vi "Write to Lights.vi"   [LabVIEW 2015]
uses:
  Common Code/Shooter State.ctl
  Common Code/Utilities/TimeManager.vi
  Common Code/Change Detect.vi
  Common Code/Change Detect Boolean.vi
  Robot Code/Robot Global Data.vi
types:
  T1 = typedef "Shooter State.ctl" = enum16{"Idle", "Warmup", "Shooter Ready", "Shoot"}
  T2 = typedef "Dashboard Display Data.ctl" = cluster{"Auton Command Cluster":T3, "Auton File Lists":T4, "Drivetrain Status Cluster":T5, "Encoder Values":T8, "IMU Data":T10, "Power and Diagnostic Data":T13, "Gyro":dbl, "Shooter State Cluster":T16, "Intake Status Cluster":T19, "Ultrasonic Data":T22, "Climb Status Cluster":T23, "Loop Times":T25}
  T3 = typedef "Auton Command Cluster.ctl" = cluster{"Command ID":i32, "maxTime":dbl, "Y Distance":dbl, "Heading":dbl, "Throttle":dbl, "Async":dbl, "Velocity":dbl, "Acceleration":dbl, "To":dbl, "Condition":dbl, "Shot Type":dbl, "Left RPM":dbl, "Override RPM":i32, "Override Angle":i32, "Right RPM":dbl, "Angle":dbl, "Intake Mode":i32, "Intake Cmd":i32, "Intake O":i32, "Eject O":i32, "Angle O":i32, "Arm O":i32, "Intake Speed":dbl, "Eject Speed":dbl, "Arm Angle":dbl, "Arm Speed":dbl, "Intake?":i32, "Eject?":i32}
  T4 = typedef "Auton File Lists.ctl" = cluster{"Current Queue":string, "General Scripts":string, "Defense Scripts":string, "Movement Scripts":string}
  T5 = typedef "Drivetrain Status Cluster.ctl" = cluster{"Modes":T6, "Y (Throttle)":dbl, "X (Steer)":dbl, "Gyro In Range?":bool, "Distance Drive Finished?":bool, "Stop Eject Lockout":bool, "Dist Drive Status":T7, "Y Target":dbl, "Heading Target":dbl, "Vision Target Aligned?":bool, "Gear":dbl, "1st Gear Time":dbl, "2nd Gear Time":dbl, "1st Gear Shifts":dbl, "2nd Gear Shifts":dbl}
  T6 = typedef "Drivetrain Modes.ctl" = enum16{"Tank", "Climb", "Manual", "Ball Vision Targeting", "Goal Vision Targeting", "PID Distance Drive", "Hybrid"}
  T7 = typedef "Dist Drive Status.ctl" = cluster{"Y In Range":bool, "X In Range":bool, "Gyro In Range":bool, "Y Dist":dbl, "X Dist":dbl, "Gyro":dbl}
  T8 = typedef "Encoder Values Super Cluster.ctl" = cluster{"Left Encoder":T9, "Right Encoder":T9}
  T9 = typedef "Encoder Values.ctl" = cluster{"Distance":dbl, "Speed":dbl, "Ticks":dbl}
  T10 = typedef "IMU Data.ctl" = cluster{"Pitch":sgl, "Roll":sgl, "Yaw":sgl, "Data Valid?":bool, "Temp":sgl, "MOVING":bool, "YAW_STABLE":bool, "Accel X":sgl, "Accel Y":sgl, "Accel Z":sgl, "Accel Magnitude":sgl, "Pitch Rate":sgl, "Roll Rate":sgl, "Yaw Rate":sgl, "NavX Opened?":bool, "NAVX_CAL_STATUS":T11, "NAVX_OP_STATUS":T12}
  T11 = typedef "navX-MXP IMU.lvlib/navX NAVX_CAL_STATUS.ctl" = u8
  T12 = typedef "navX-MXP IMU.lvlib/navX NAVX_OP_STATUS.ctl" = u8
  T13 = typedef "Power and Diagnostic Data.ctl" = cluster{"PDP Data":T14, "PCM Data":T15, "roboRIO input voltage (V)":dbl, "roboRIO input current (A)":dbl, "3.3V Rail Short":bool, "5 V Rail Short":bool, "6 V Rail Short":bool, "roboRIO Brownout":bool, "Outputs Enabled?":bool}
  T14 = typedef "PDP Data.ctl" = cluster{"Battery Voltage":sgl, "Temperature (degrees C)":sgl, "Internal Battery R (Ohms)":sgl, "Energy (J)":sgl, "Power (W)":sgl, "Total Current (A)":sgl, "Battery Voltage Fault":bool, "Temperature Fault":bool, "Hardware Fault":bool, "Currents":cluster{"[0]":sgl, "[1]":sgl, "[2]":sgl, "[3]":sgl, "[4]":sgl, "[5]":sgl, "[6]":sgl, "[7]":sgl, "[8]":sgl, "[9]":sgl, "[10]":sgl, "[11]":sgl, "[12]":sgl, "[13]":sgl, "[14]":sgl, "[15]":sgl}, "Current Faults":cluster{"[0]":bool, "[1]":bool, "[2]":bool, "[3]":bool, "[4]":bool, "[5]":bool, "[6]":bool, "[7]":bool, "[8]":bool, "[9]":bool, "[10]":bool, "[11]":bool, "[12]":bool, "[13]":bool, "[14]":bool, "[15]":bool}}
  T15 = typedef "PCM Data.ctl" = cluster{"Compressor Fault":bool, "Solenoid Fault":bool, "Compressor Enabled":bool, "Hardware Fault":bool, "Compressor Current":dbl}
  T16 = typedef "Shooter State Cluster.ctl" = cluster{"State":T1, "Left RPM":dbl, "Right RPM":dbl, "Shooter Ready?":bool, "Ball Loaded?":bool, "Current Angle":dbl, "Angle Motor Output":dbl, "Trigger Output":dbl, "Angle Ready?":bool, "RPM Ready?":bool, "Vision Ready?":bool, "Ball Loaded?":bool, "Mode":T17, "Shot Type":T18, "Pot Height":dbl, "Current Tripped Forward?":bool, "Current Tripped Backward?":bool, "Right Servo":i32, "Left Servo":i32, "IR Override":bool, "Intake Danger?":bool}
  T17 = typedef "Shoot Modes Enum.ctl" = enum16{"Manual", "Safe", "Auto"}
  T18 = typedef "Shot Type.ctl" = enum16{"Batter Shot", "Corner Shot", "Curve Shot", "Vision Shot", "Deep Middle Shot"}
  T19 = typedef "Intake Status Cluster.ctl" = cluster{"Roller Power":dbl, "Angle Power":dbl, "Intake Mode":T20, "Intake States":T21, "Rollers Active?":bool, "Current Height":dbl, "Target Height":dbl, "Encoder Raw Position":dbl, "Forward Tripped?":bool, "Backward Tripped?":bool, "Override IR?":bool}
  T20 = typedef "Intake Mode.ctl" = enum16{"Safe", "Auto", "Manual"}
  T21 = typedef "Intake States.ctl" = enum16{"Idle", "Set roller speed", "Move to angle"}
  T22 = typedef "Ultrasonic Data.ctl" = cluster{"Left Ultrasonic":dbl, "Right Ultrasonic":dbl}
  T23 = typedef "Climb Status Cluster.ctl" = cluster{"Pull Power":dbl, "Unpin Power":dbl, "PTO Engaged?":bool, "Pull Height":dbl, "Climb Mode":T24}
  T24 = typedef "Climb Mode.ctl" = enum16{"Auto", "Manual"}
  T25 = typedef "Major Loop Times.ctl" = cluster{"DT Loop Timer":u32, "Shooter Loop Timer":u32, "Intake Loop Timer":u32, "US Loop Timer":u32, "Auton File Loop Timer":u32}
  T26 = typedef "WPI_DriverStationRobotMode2.ctl" = enum16{"Autonomous Disabled", "Autonomous Enabled", "Teleop Disabled", "Teleop Enabled", "Disconnected", "Finish", "Test Disabled", "Test Enabled", "Emergency Stopped"}
  T27 = typedef "WPI_AOChannelDevRef.ctl" = cluster{"DevStatus":errorcluster, "AO Channel":T28}
  T28 = typedef "WPI_AnalogOutputChannel.ctl" = enum8{"AO MXP 0", "AO MXP 1", "Invalid"}
  T29 = typedef "WPI_DigitalOutputDevRef.ctl" = cluster{"DIO Channel":T30, "DevStatus":errorcluster}
  T30 = typedef "FPGA_DIOChannel.ctl" = enum8{"DIO 0", "DIO 1", "DIO 2", "DIO 3", "DIO 4", "DIO 5", "DIO 6", "DIO 7", "DIO 8", "DIO 9", "DIO MXP 0", "DIO MXP 1", "DIO MXP 2", "DIO MXP 3", "DIO MXP 4", "DIO MXP 5", "DIO MXP 6", "DIO MXP 7", "DIO MXP 8", "DIO MXP 9", "DIO MXP 10", "DIO MXP 11", "DIO MXP 12", "DIO MXP 13", "DIO MXP 14", "DIO MXP 15", "Invalid"}
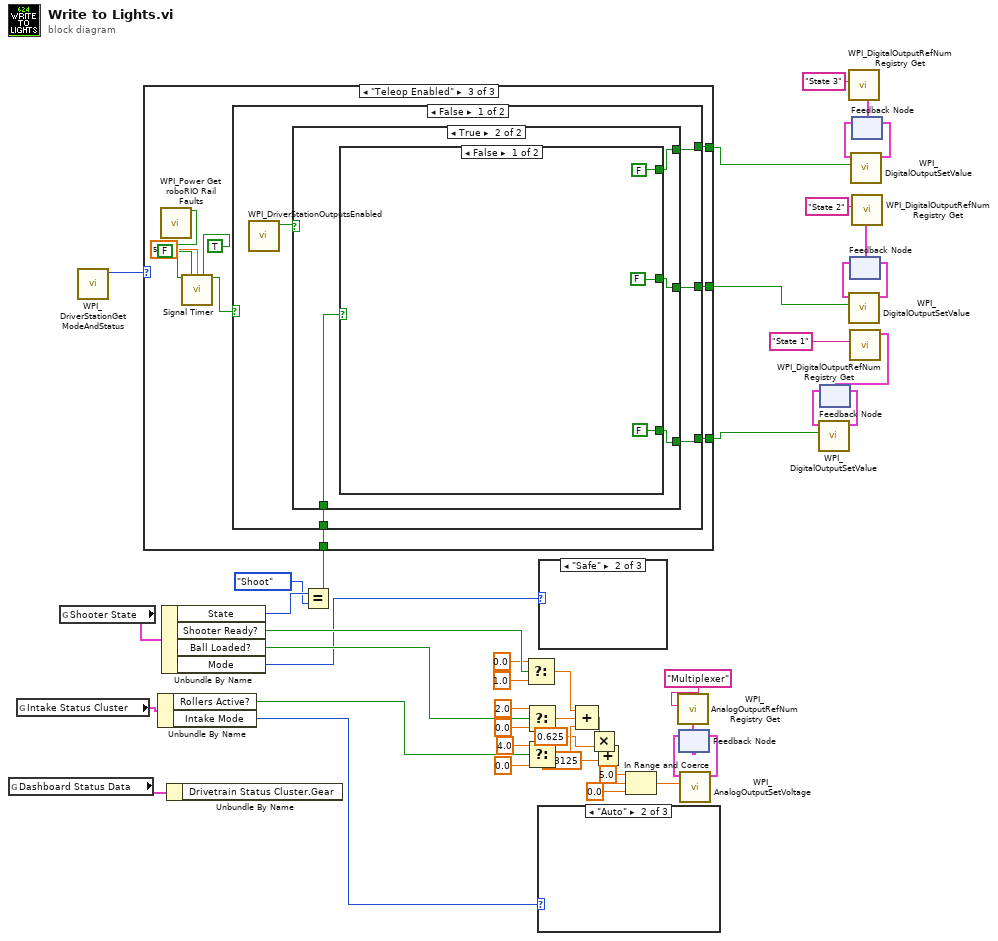
[diagram p0: block diagram]
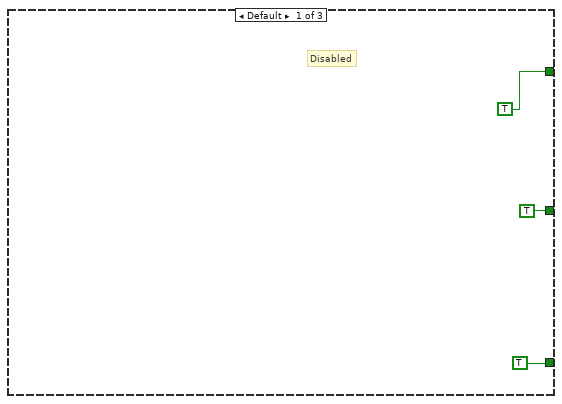
[diagram p6: hidden frame]
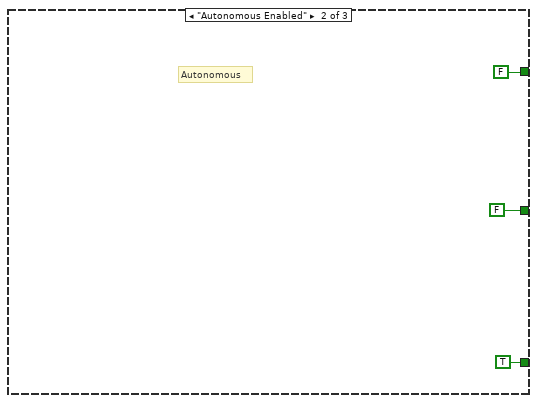
[diagram p7: hidden frame]
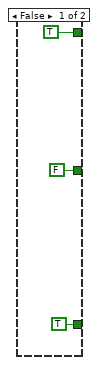
[diagram p8: hidden frame]
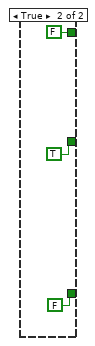
[diagram p9: hidden frame]
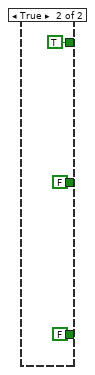
[diagram p10: hidden frame]
diagram:
  n1 = global read "Robot Global Data.vi" "Dashboard Status Data"() -> (w27:T2)
  n2 = global read "Robot Global Data.vi" "Intake Status Cluster"() -> (w28:T19)
  n3 = global read "Robot Global Data.vi" "Shooter State"() -> (w32:T16)
  n4 = call <vilib>:"WPI_DriverStationGetModeAndStatus.vi"() -> ("Robot Mode"=w36:T26)  [unwired: 10 in, 1 out]
  n5 = Unbundle By Name(w28) -> ("Rollers Active?"=w16:bool, "Intake Mode"=w1:T20)
  n6 = Unbundle By Name(w32) -> ("State"=w31:T1, "Shooter Ready?"=w13:bool, "Ball Loaded?"=w15:bool, "Mode"=w2:T17)
  n7 = Unbundle By Name(w27) -> ()  [unwired: 1 out]
  n8 = Equal?(x=w31, y=Shooter_State."Shoot") -> (x = y?=w29:bool)
  n9 = case shown="\"Teleop Enabled\"" w36 {
    tunnel: [TRUE FALSE w63] -> w33
    tunnel: [TRUE FALSE w62] -> w34
    tunnel: [TRUE TRUE w61] -> w35
    tunnel: w29 -> [_ _ w55]
    frame Default {
      # "Disabled"
    }
    frame "Autonomous Enabled" {
      # "Autonomous"
    }
    frame "Teleop Enabled" {
      n10 = call <vilib>:"WPI_Power Get roboRIO Rail Faults.vi"() -> ("Input Voltage Brown Out"=w60:bool)  [unwired: 10 in, 5 out]
      n11 = call "Signal Timer.vi"("Input"=w60, "Edge"=FALSE, "Interval"=500.0, "Pull"=TRUE) -> ("Filtered Output"=w56:bool)  [unwired: 11 in]
      n12 = case shown="False" w56 {
        tunnel: [w67 TRUE] -> w63
        tunnel: [w66 FALSE] -> w62
        tunnel: [w65 FALSE] -> w61
        tunnel: w55 -> [w64 _]
        frame False {
          n13 = call <vilib>:"WPI_DriverStationOutputsEnabled.vi"() -> ("OutputsEnabled?"=w68:bool)  [unwired: 10 in, 1 out]
          n14 = case shown="True" w68 {
            tunnel: [TRUE w74] -> w67
            tunnel: [FALSE w73] -> w66
            tunnel: [TRUE w72] -> w65
            tunnel: w64 -> [_ w75]
            frame False {
            }
            frame True {
              n15 = case shown="False" w75 {
                tunnel: [FALSE FALSE] -> w74
                tunnel: [FALSE TRUE] -> w73
                tunnel: [FALSE FALSE] -> w72
                frame False {
                }
                frame True {
                }
              }
            }
          }
        }
        frame True {
        }
      }
    }
  }
  n16 = Select(t=0.0, s=w13, f=1.0) -> (s? t:f=w14:dbl)
  n17 = Select(t=2.0, s=w15, f=0.0) -> (s? t:f=w18:dbl)
  n18 = Select(t=4.0, s=w16, f=0.0) -> (s? t:f=w17:dbl)
  n19 = case shown="\"Auto\"" w1 {
    frame "Safe", Default {
    }
    frame "Auto" {
    }
    frame "Manual" {
    }
  }
  n20 = case shown="\"Safe\"" w2 {
    frame "Manual", Default {
    }
    frame "Safe" {
    }
    frame "Auto" {
    }
  }
  n21 = Compound Arithmetic op=ADD(w14, w18, w17) -> (w22:dbl)
  n22 = Multiply(x=w22, y=0.625) -> (x*y=w6:dbl)
  n23 = Add(x=w6, y=0.3125) -> (x+y=w4:dbl)
  n24 = In Range and Coerce(upper limit=5.0, x=w4, lower limit=0.0) -> (coerced(x)=w21:dbl)  [unwired: 1 out]
  n25 = call <vilib>:"WPI_AnalogOutputRefNum Registry Get.vi"("refnum name"="Multiplexer") -> ("AODeviceRef"=w24:T27)  [unwired: 9 in, 1 out]
  n26 = feedback #1(w24) -> (w25:T27)
  n27 = call <vilib>:"WPI_AnalogOutputSetVoltage.vi"("Voltage"=w21, "AODeviceRef"=w25) -> ("AODeviceRef"=w23:T27)  [unwired: 8 in, 1 out]
  n28 = feedback-in #1(w23) -> ()
  n29 = call <vilib>:"WPI_DigitalOutputRefNum Registry Get.vi"("refnum name"="State 3") -> ("DigitalOutputDevRef"=w41:T29)  [unwired: 9 in, 1 out]
  n30 = call <vilib>:"WPI_DigitalOutputRefNum Registry Get.vi"("refnum name"="State 1") -> ("DigitalOutputDevRef"=w37:T29)  [unwired: 9 in, 1 out]
  n31 = feedback #2(w37) -> (w46:T29)
  n32 = call <vilib>:"WPI_DigitalOutputSetValue.vi"("Value"=w35, "DigitalOutputDevRef"=w46) -> ("DigitalOutputDevRef"=w47:T29)  [unwired: 8 in, 1 out]
  n33 = feedback-in #2(w47) -> ()
  n34 = feedback #3(w41) -> (w40:T29)
  n35 = call <vilib>:"WPI_DigitalOutputSetValue.vi"("Value"=w33, "DigitalOutputDevRef"=w40) -> ("DigitalOutputDevRef"=w38:T29)  [unwired: 8 in, 1 out]
  n36 = feedback-in #3(w38) -> ()
  n37 = call <vilib>:"WPI_DigitalOutputRefNum Registry Get.vi"("refnum name"="State 2") -> ("DigitalOutputDevRef"=w42:T29)  [unwired: 9 in, 1 out]
  n38 = feedback #4(w42) -> (w44:T29)
  n39 = call <vilib>:"WPI_DigitalOutputSetValue.vi"("Value"=w34, "DigitalOutputDevRef"=w44) -> ("DigitalOutputDevRef"=w43:T29)  [unwired: 8 in, 1 out]
  n40 = feedback-in #4(w43) -> ()
